vi "Get Robot Competition Mode.vi"(10 "Finish":bool, 11 "DS Occurrence":refnum<k4>) -> (0 "Match Info out":T1={"Autonomous Elapsed Seconds"=0.0, "TeleOp Elapsed Seconds"=0.0, "Disabled Elapsed Seconds"=0.0, "Visited Autonomous"=FALSE, "Visited TeleOp"=FALSE, "Visited Disabled"=FALSE, "Autonomous Settings"={"Autonomous Style"=enum."Independent", "VI Refnum"=refnum}}, 1 "RawControlByte":u8 format="%08b", 2 "Call Context":T2, 3 "Robot Mode":T3)   [LabVIEW 2013]
doc: "<b>Get Competition Mode.vi</b> returns the mode of the current phase of competition, which determines the current restrictions of robot operation that apply. Possible modes include <b>Autonomous Disabled</b>, <b>Autonomous Enabled</b>, <b>Teleop Disabled</b>, and <b>Teleop Enabled</b>.\n\nThis software is licensed. Open the labview\\readme\\WPI Robotics Library Open Source License.txt file for more information."
uses:
  <vilib>/Rock Robotics/WPI/DriverStation/WPI_DriverStationRobotMode.ctl
  <vilib>/Rock Robotics/WPI/DriverStation/WPI_DriverStationDerivedRobotMode.ctl
  <vilib>/Rock Robotics/WPI/DriverStation/WPI_DriverStationMatch Info.ctl
  <vilib>/Rock Robotics/WPI/DriverStation/WPI_DriverStationCommDataCacheOp.ctl
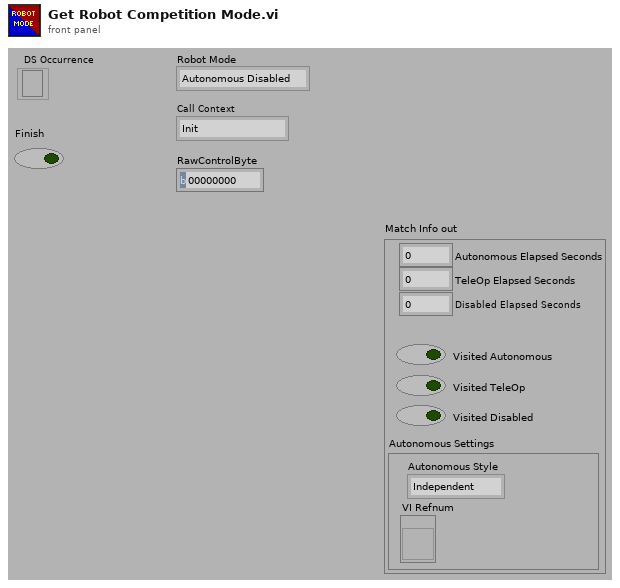
[diagram p1: front panel]
types:
  T1 = typedef "WPI_DriverStationMatch Info.ctl" = cluster{"Autonomous Elapsed Seconds":dbl, "TeleOp Elapsed Seconds":dbl, "Disabled Elapsed Seconds":dbl, "Visited Autonomous":bool, "Visited TeleOp":bool, "Visited Disabled":bool, "Autonomous Settings":cluster{"Autonomous Style":enum16{"Iterative", "Independent"}, "VI Refnum":refnum<vi>}}
  T2 = typedef "WPI_DriverStationDerivedRobotMode.ctl" = enum16{"Init", "Execute", "Stop"}
  T3 = typedef "WPI_DriverStationRobotMode.ctl" = enum16{"Autonomous Disabled", "Autonomous Enabled", "Teleop Disabled", "Teleop Enabled", "Timeout", "Finish"}
  T4 = typedef "WPI_DriverStationCommDataCacheOp.ctl" = enum16{"Get", "Set", "Init"}
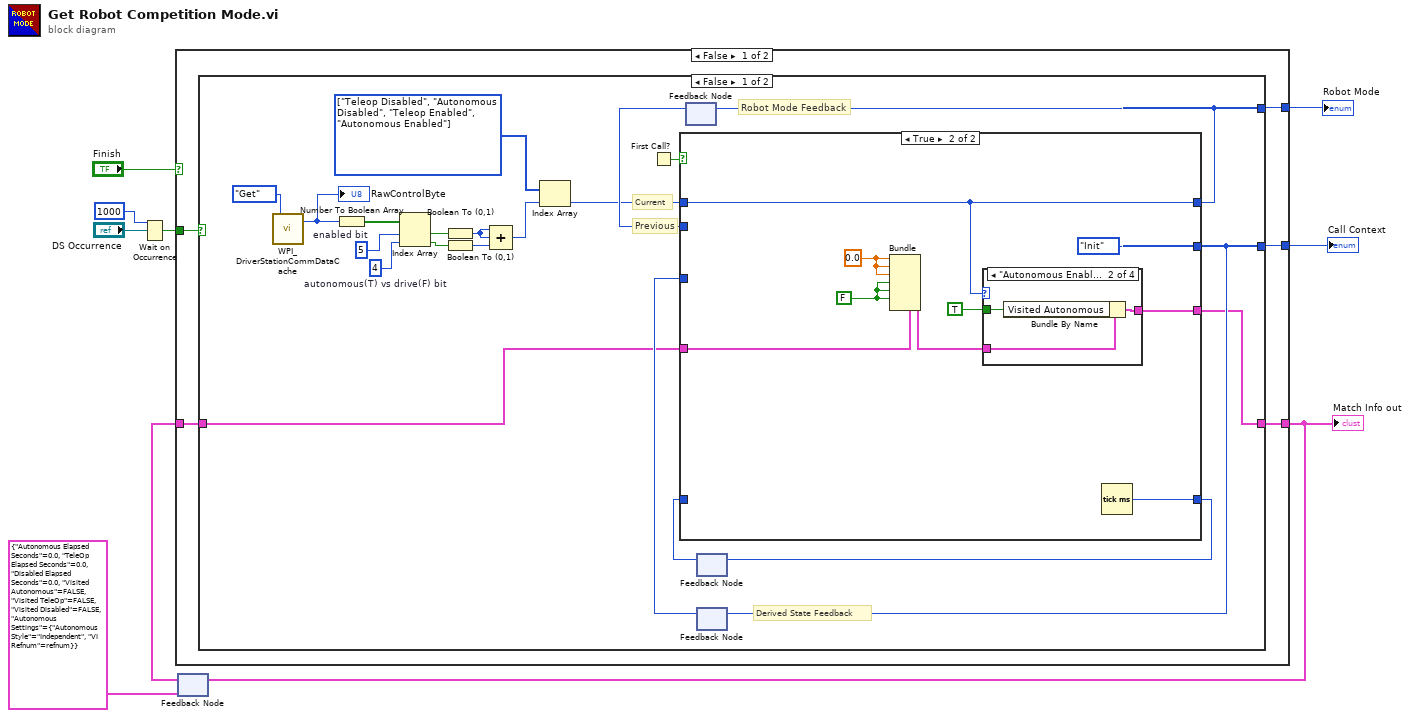
[diagram p0: block diagram]
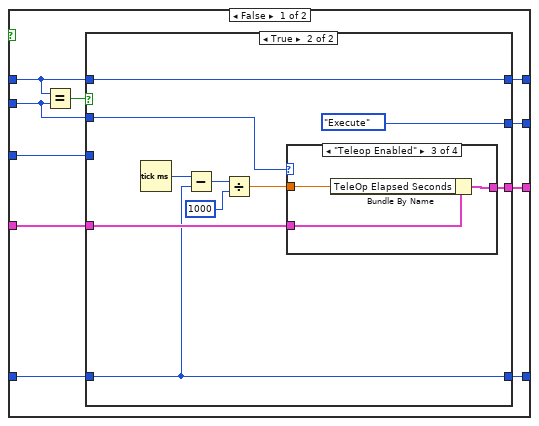
[diagram p2: hidden frame]
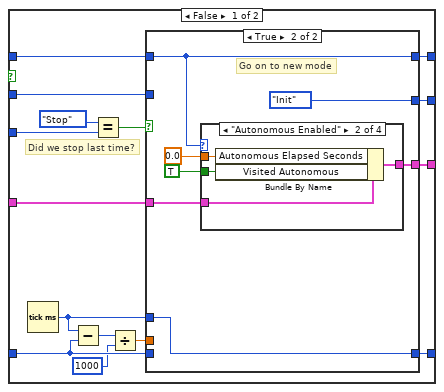
[diagram p3: hidden frame]
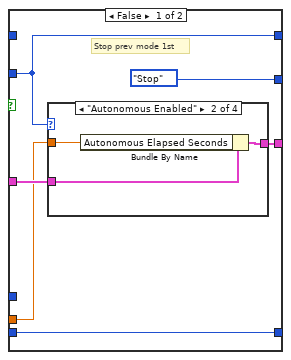
[diagram p4: hidden frame]
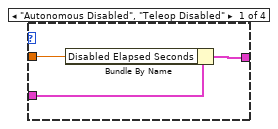
[diagram p5: hidden frame]
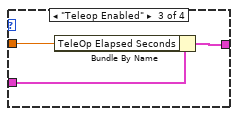
[diagram p6: hidden frame]
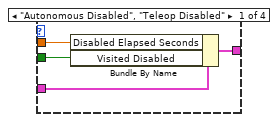
[diagram p8: hidden frame]
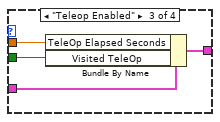
[diagram p9: hidden frame]
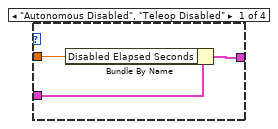
[diagram p11: hidden frame]
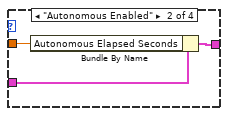
[diagram p12: hidden frame]
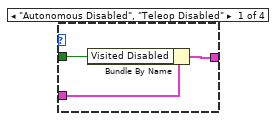
[diagram p14: hidden frame]
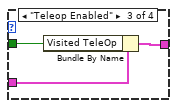
[diagram p15: hidden frame]
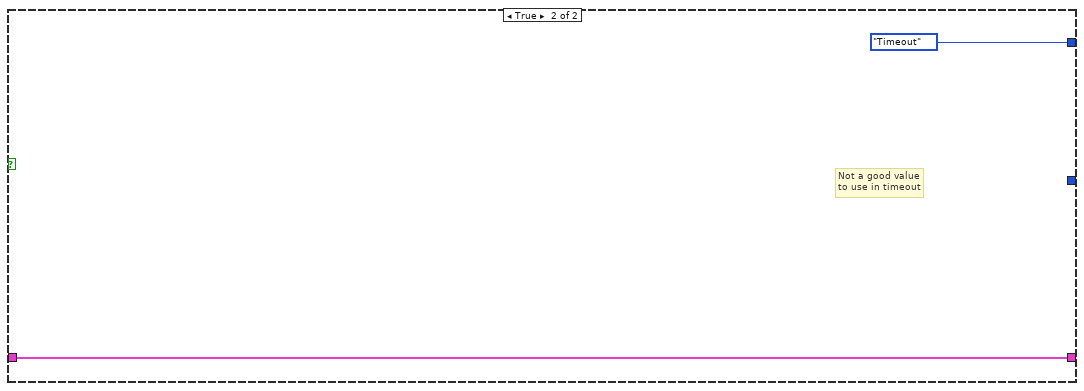
[diagram p17: hidden frame]
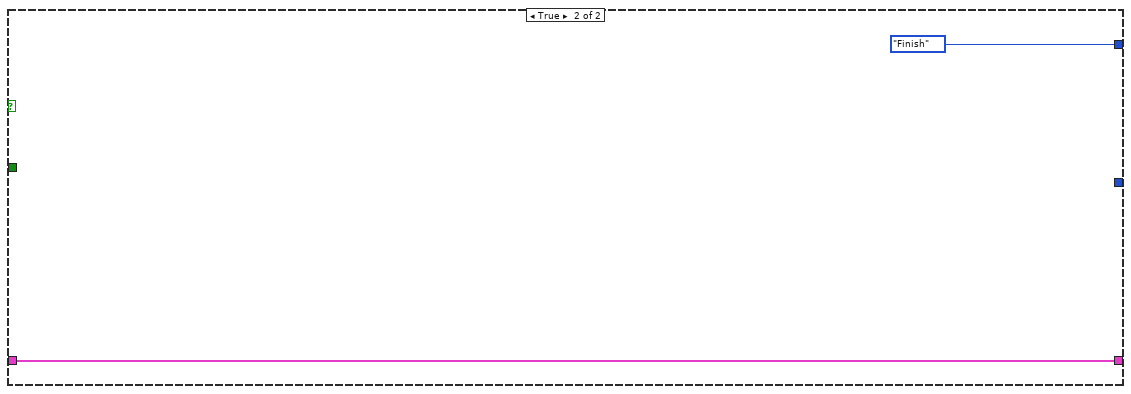
[diagram p18: hidden frame]
diagram:
  n1 = Wait on Occurrence(2:"DS Occurrence", 3:1000 ("ms timeout (-1)")) -> (0:w6:bool)  [unwired: 1 out]
  n2 = feedback #1(T1 {"Autonomous Elapsed Seconds"=0.0, "TeleOp Elapsed Seconds"=0.0, "Disabled Elapsed Seconds"=0.0, "Visited Autonomous"=FALSE, "Visited TeleOp"=FALSE, "Visited Disabled"=FALSE, "Autonomous Settings"={"Autonomous Style"=enum."Independent", "VI Refnum"=refnum}} ("Match Info")) -> (w2:T1)
  n3 = case shown="False" "Finish" {
    tunnel: [w14 _] -> w9
    tunnel: [w13 WPI_DriverStationRobotMode."Finish" ("RobotMode")] -> w8
    tunnel: w6 -> [w12 _]
    tunnel: w2 -> [w11 w138]
    tunnel: [w10 w138] -> w3
    frame False {
      n4 = case shown="False" w12 {
        tunnel: [w27 _] -> w14
        tunnel: [w26 WPI_DriverStationRobotMode."Timeout" ("RobotMode")] -> w13
        tunnel: w11 -> [w15 w136]
        tunnel: [w16 w136] -> w10
        frame False {
          w25 = T3[] [enum."Teleop Disabled", enum."Autonomous Disabled", enum."Teleop Enabled", enum."Autonomous Enabled"] items=["Autonomous Disabled", "Autonomous Enabled", "Teleop Disabled", "Teleop Enabled", "Timeout", "Finish"]
          w31 = 4  # autonomous(T) vs drive(F) bit
          w32 = 5  # enabled bit
          # "Derived State Feedback"
          # "Robot Mode Feedback"
          # "Previous"
          # "Current"
          n5 = call <vilib>:"WPI_DriverStationCommDataCache.vi"("CommDataCacheOp"=WPI_DriverStationCommDataCacheOp."Get") -> ("ControlBit out"=w34:u8)  [unwired: 18 out]
          "RawControlByte" <- w34
          n6 = Number To Boolean Array(number=w34) -> (Boolean array=w33:bool[])
          n7 = Index Array(array=w33, index #1=w32, index #2=w31) -> (element #1=w22:bool, element #2=w21:bool)
          n8 = Boolean To (0,1)(Boolean=w22) -> (0, 1=w24:i16)
          n9 = Boolean To (0,1)(Boolean=w21) -> (0, 1=w23:i16)
          n10 = Compound Arithmetic op=ADD(w24, w24, w23) -> (w20:i16)
          n11 = Index Array(array=w25, index=w20) -> (element=w19:T3)
          n12 = First Call?() -> (First Call?: T/F=w28:bool)
          n13 = feedback #2() -> (w29:T3)  [unwired: 1 out]
          n14 = feedback #3() -> (w17:u32)  [unwired: 1 out]
          n15 = feedback #4() -> (w30:T2)  [unwired: 1 out]
          n16 = case shown="True" w28 {
            tunnel: [w45 w117] -> w26
            tunnel: [w44 WPI_DriverStationDerivedRobotMode."Init" ("Derived Robot State")] -> w27
            tunnel: w30 -> [w42 _]
            tunnel: w19 -> [w41 w117]
            tunnel: w29 -> [w40 _]
            tunnel: w15 -> [w39 w124]
            tunnel: [w38 w119] -> w16
            tunnel: [w36 w121] -> w18
            tunnel: w17 -> [w37 _]
            frame False {
              n17 = Equal?(x=w41, y=w40) -> (x = y?=w43:bool)
              n18 = case shown="True" w43 {
                tunnel: w41 -> [w58 w106]
                tunnel: [w57 w106] -> w45
                tunnel: [w56 WPI_DriverStationDerivedRobotMode."Execute" ("Derived Robot State")] -> w44
                tunnel: w42 -> [w60 _]
                tunnel: w40 -> [w55 w101]
                tunnel: w39 -> [w49 w102]
                tunnel: [w53 w103] -> w38
                tunnel: w37 -> [w50 w100]
                tunnel: [w51 w100] -> w36
                frame False {
                  # "Did we stop last time?"
                  n19 = Tick Count (ms)() -> (millisecond timer value=w52:u32)
                  n20 = Subtract(x=w52, y=w50) -> (x-y=w48:u32)
                  n21 = Equal?(x=WPI_DriverStationDerivedRobotMode."Stop" ("Derived Robot State"), y=w60) -> (x = y?=w59:bool)
                  n22 = Divide(x=w48, y=1000) -> (x/y=w47:dbl)
                  n23 = case shown="True" w59 {
                    tunnel: w58 -> [_ w82]
                    tunnel: [w61 w82] -> w57
                    tunnel: [WPI_DriverStationDerivedRobotMode."Stop" ("Derived Robot State") WPI_DriverStationDerivedRobotMode."Init" ("Derived Robot State")] -> w56
                    tunnel: w55 -> [w61 _]
                    tunnel: w49 -> [w64 w80]
                    tunnel: [w65 w79] -> w53
                    tunnel: w47 -> [w63 _]
                    tunnel: w52 -> [_ w77]
                    tunnel: [w62 w77] -> w51
                    tunnel: w50 -> [w62 _]
                    frame False {
                      # "Stop prev mode 1st"
                      n24 = case shown="\"Autonomous Enabled\"" w61 {
                        tunnel: w63 -> [w69 w72 w75 _]
                        tunnel: w64 -> [w68 w71 w74 w76]
                        tunnel: [w67 w70 w73 w76] -> w65
                        frame "Autonomous Disabled", "Teleop Disabled" {
                          n25 = Bundle By Name(cluster=w68, "Disabled Elapsed Seconds"=w69) -> (w67:T1)
                        }
                        frame "Autonomous Enabled" {
                          n26 = Bundle By Name(cluster=w71, "Autonomous Elapsed Seconds"=w72) -> (w70:T1)
                        }
                        frame "Teleop Enabled" {
                          n27 = Bundle By Name(cluster=w74, "TeleOp Elapsed Seconds"=w75) -> (w73:T1)
                        }
                        frame Default {
                        }
                      }
                    }
                    frame True {
                      # "Go on to new mode"
                      n28 = case shown="\"Autonomous Enabled\"" w82 {
                        tunnel: 0.0 -> [w87 w91 w92 _]
                        tunnel: w80 -> [w86 w90 w95 w96]
                        tunnel: [w85 w89 w94 w96] -> w79
                        tunnel: TRUE -> [w84 w88 w93 _]
                        frame "Autonomous Disabled", "Teleop Disabled" {
                          n29 = Bundle By Name(cluster=w86, "Disabled Elapsed Seconds"=w87, "Visited Disabled"=w84) -> (w85:T1)
                        }
                        frame "Autonomous Enabled" {
                          n30 = Bundle By Name(cluster=w90, "Autonomous Elapsed Seconds"=w91, "Visited Autonomous"=w88) -> (w89:T1)
                        }
                        frame "Teleop Enabled" {
                          n31 = Bundle By Name(cluster=w95, "TeleOp Elapsed Seconds"=w92, "Visited TeleOp"=w93) -> (w94:T1)
                        }
                        frame Default {
                        }
                      }
                    }
                  }
                }
                frame True {
                  n32 = Tick Count (ms)() -> (millisecond timer value=w104:u32)
                  n33 = Subtract(x=w104, y=w100) -> (x-y=w98:u32)
                  n34 = Divide(x=w98, y=u32 1000) -> (x/y=w99:dbl)
                  n35 = case shown="\"Teleop Enabled\"" w101 {
                    tunnel: w99 -> [w109 w112 w115 _]
                    tunnel: w102 -> [w108 w111 w114 w116]
                    tunnel: [w107 w110 w113 w116] -> w103
                    frame "Autonomous Disabled", "Teleop Disabled" {
                      n36 = Bundle By Name(cluster=w108, "Disabled Elapsed Seconds"=w109) -> (w107:T1)
                    }
                    frame "Autonomous Enabled" {
                      n37 = Bundle By Name(cluster=w111, "Autonomous Elapsed Seconds"=w112) -> (w110:T1)
                    }
                    frame "Teleop Enabled" {
                      n38 = Bundle By Name(cluster=w114, "TeleOp Elapsed Seconds"=w115) -> (w113:T1)
                    }
                    frame Default {
                    }
                  }
                }
              }
            }
            frame True {
              w123 = 0.0
              w122 = FALSE
              n39 = Bundle(cluster=w124, "Autonomous Elapsed Seconds"=w123, "TeleOp Elapsed Seconds"=w123, "Disabled Elapsed Seconds"=w123, "Visited Autonomous"=w122, "Visited TeleOp"=w122, "Visited Disabled"=w122) -> (w120:T1)  [unwired: 1 out]
              n40 = case shown="\"Autonomous Enabled\"" w117 {
                tunnel: w120 -> [w128 w131 w134 w135]
                tunnel: [w127 w130 w133 w135] -> w119
                tunnel: TRUE -> [w126 w129 w132 _]
                frame "Autonomous Disabled", "Teleop Disabled" {
                  n41 = Bundle By Name(cluster=w128, "Visited Disabled"=w126) -> (w127:T1)
                }
                frame "Autonomous Enabled" {
                  n42 = Bundle By Name(cluster=w131, "Visited Autonomous"=w129) -> (w130:T1)
                }
                frame "Teleop Enabled" {
                  n43 = Bundle By Name(cluster=w134, "Visited TeleOp"=w132) -> (w133:T1)
                }
                frame Default {
                }
              }
              n44 = Tick Count (ms)() -> (millisecond timer value=w121:u32)
            }
          }
          n45 = feedback-in #2(w26) -> ()
          n46 = feedback-in #3(w18) -> ()
          n47 = feedback-in #4(w27) -> ()
        }
        frame True {
          # "Not a good value\nto use in timeout"
        }
      }
    }
    frame True {
    }
  }
  "Robot Mode" <- w8
  "Call Context" <- w9
  "Match Info out" <- w3
  n48 = feedback-in #1(w3) -> ()
